vi "sendNotifierStopServer.vi"(8 "error in (no error)":errorcluster, 11 "TcpServerCmd in":refnum<class "TcpServerCmd.lvclass">) -> (0 "error out":errorcluster, 3 "TcpServerCmd out":refnum<class "TcpServerCmd.lvclass">)   [LabVIEW 2018, in "TcpServerCmd.lvclass"]
doc: "Send the notifierStopServer to stop the runServer.vi."
uses:
  TcpServerCmd.lvclass
  home/pcortes/Documents/github/ts_labview_tcp_json/src/TcpServerBase/TcpServerBase.lvclass
  TcpServerBase/TcpServerBase.lvclass
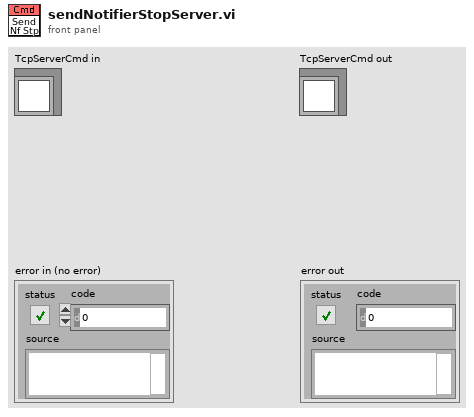
[diagram p1: front panel]
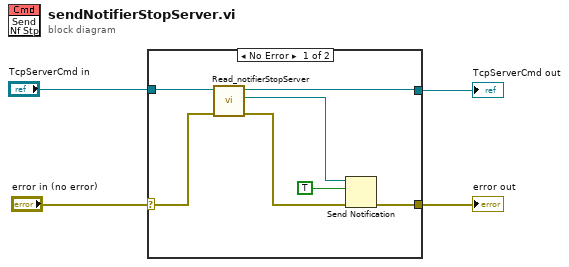
[diagram p0: block diagram]
diagram:
  n1 = case shown="No Error" "error in (no error)" {
    selector: "error in (no error)" -> [w6 w13]
    tunnel: "TcpServerCmd in" -> [w11 w12]
    tunnel: [w10 w13] -> w2
    tunnel: [w8 w12] -> w1
    frame No Error {
      n2 = call "Read_notifierStopServer.vi"("error in (no error)"=w6, "TcpServerBase in"=w11) -> ("error out"=w5:errorcluster, "notifierStopServer"=w7:refnum<notifier>, "TcpServerBase out"=w8:refnum<class "TcpServerCmd.lvclass">)  [unwired: 7 in]
      n3 = Send Notification(notification=TRUE, notifier=w7, error in (no error)=w5) -> (error out=w10:errorcluster)  [unwired: 1 out]
    }
    frame Error {
    }
  }
  "error out" <- w2
  "TcpServerCmd out" <- w1
